vi "Design Challenge Steph.vi"() -> ()   [LabVIEW 2025]
panel:
  out "Initial Height (m)":dbl(slide) scale=0.0..100.0
  out "Trajectory":cluster{"X":dbl, "Y":dbl}[](graph)
  in  "theta_initial":dbl
  in  "V_initial (m/s)":dbl
  in  "Mass (kg)":dbl
  # "FIVE NIGHTS AT  LABVIEW"
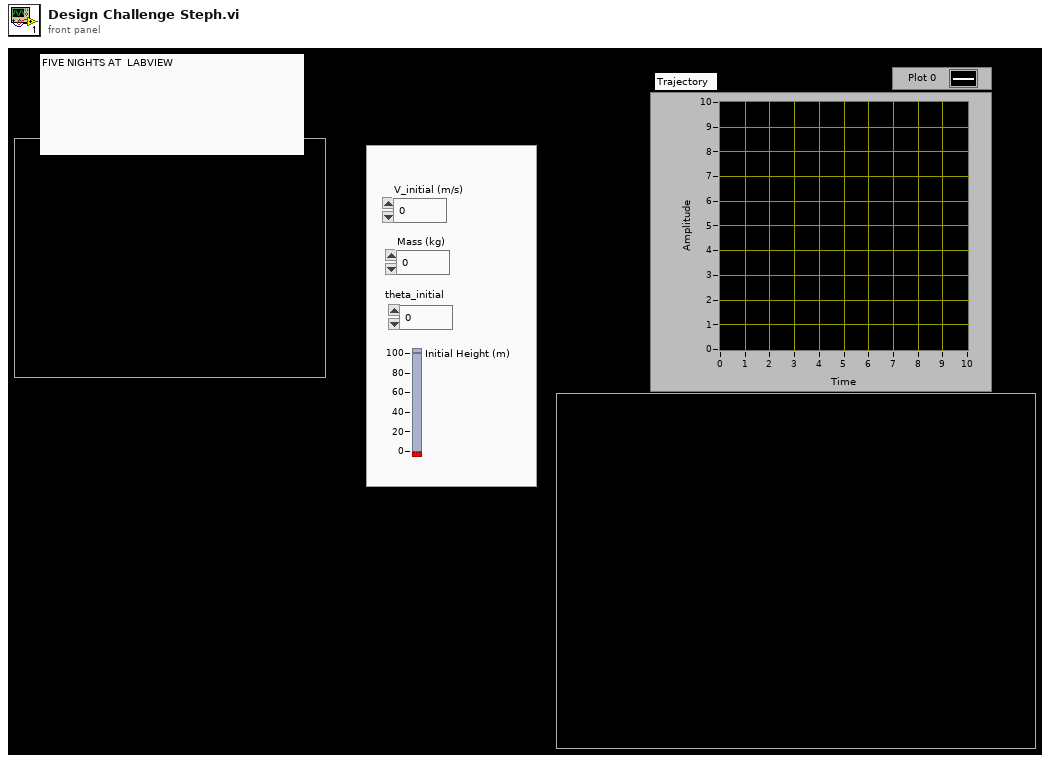
[diagram p1: front panel]
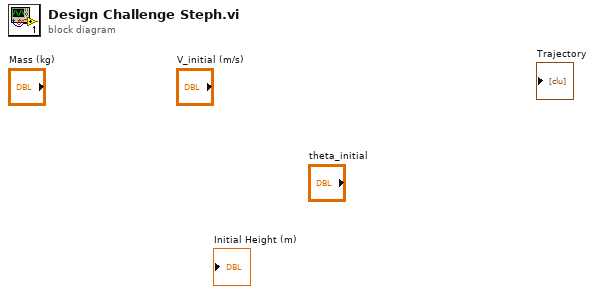
[diagram p0: block diagram]
diagram:
